vi "client.vi"() -> ()   [LabVIEW 2016]
panel:
  in  "values to send":string[](array[string])
  out "echoed values":string[](array[string])
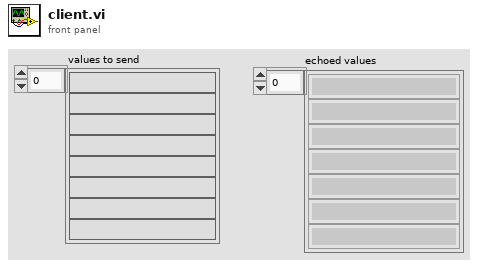
[diagram p1: front panel]
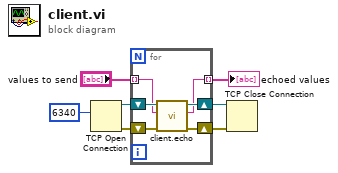
[diagram p0: block diagram]
diagram:
  n1 = TCP Open Connection(remote port or service name=u16 6340) -> (connection ID=w6:refnum<k5>, error out=w5:errorcluster)  [unwired: 4 in]
  n2 = for {
    tunnel: "values to send" -> [w11] mode=indexing
    tunnel: [w9] -> w2 mode=indexing
    shift-right: [w10] -> w3
    shift-left: w6 -> [w13]
    shift-right: [w8] -> w1
    shift-left: w5 -> [w12]
    n3 = call "client.echo.vi"("error in (no error)"=w12, "value in"=w11, "TCP Network Connection in"=w13) -> ("error out"=w8:errorcluster, "value out"=w9:string, "TCP Network Connection out"=w10:refnum<k5>)  [unwired: 6 in]
  }
  "echoed values" <- w2
  n4 = TCP Close Connection(connection ID=w3, error in (no error)=w1) -> ()  [unwired: 1 in, 2 out]
